vi "WPI_MotorControlSafetyTest.vi"   [LabVIEW 2019]
doc: "Calls the SafetyCheck VI. SafetyCheck VI needs to be called dynamically by the SafetyCheckEngine, but it already gets called statically. Wrapping it in this VI enables calling it dynamically."
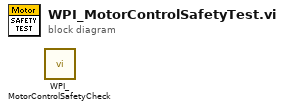
[diagram p0: block diagram]
diagram:
  n1 = call <vilib>:"WPI_MotorControlSafetyCheck.vi"() -> ()  [unwired: 3 in, 13 out]
